vi "get.Messages.vi"(8 "error in (no error)":errorcluster, 11 "SequencedUnitHeader in":refnum<class "SequencedUnitHeader.lvclass">) -> (0 "error out":errorcluster, 2 "Messages.Out":refnum<class "MessageBase.lvclass">[](array[class]), 3 "SequencedUnitHeader out":refnum<class "SequencedUnitHeader.lvclass">)   [LabVIEW 2020, in "SequencedUnitHeader.lvclass"]
uses:
  SequencedUnitHeader.lvclass
  MessageBase/MessageBase.lvclass
  SequencedUnitHeader.lvclass/SequencedUnitHeader.ctl
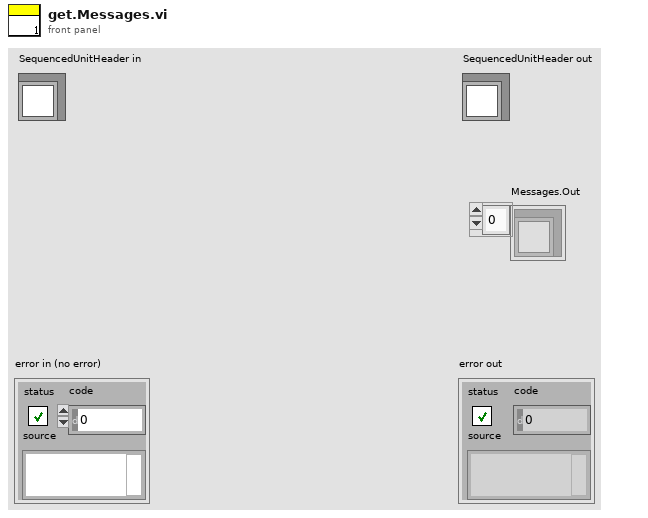
[diagram p1: front panel]
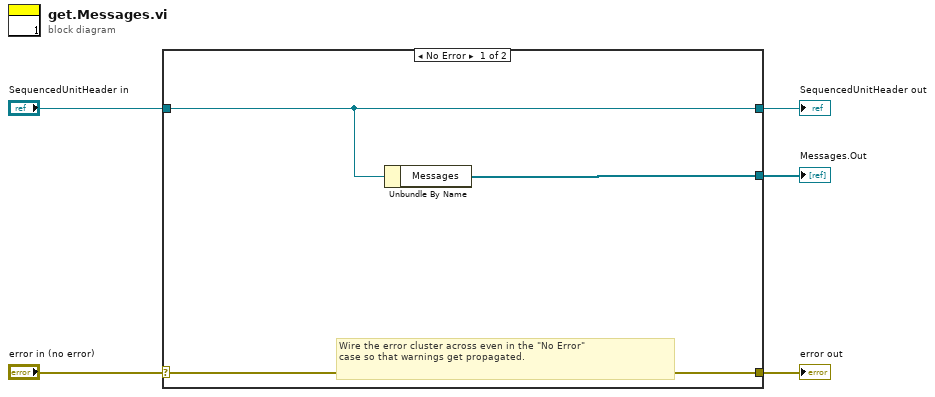
[diagram p0: block diagram]
diagram:
  n1 = case shown="No Error" "error in (no error)" {
    selector: "error in (no error)" -> [w8 w10]
    tunnel: [w8 w10] -> w4
    tunnel: [w7 w9] -> w2
    tunnel: "SequencedUnitHeader in" -> [w7 w9]
    tunnel: [w6 _] -> w1
    frame No Error {
      # "Wire the error cluster across even in the \"No Error\"\ncase so that warnings get propagated."
      n2 = Unbundle By Name(w7) -> ("Messages"=w6:refnum<class "MessageBase.lvclass">[])
    }
    frame Error {
    }
  }
  "error out" <- w4
  "SequencedUnitHeader out" <- w2
  "Messages.Out" <- w1
